vi "OAT Easy Resample Order Spectrum.vi"   [LabVIEW 2017]
doc: "Computes the order spectrum as power versus orders for <B>scaled signal [EU]</B>. You can use this polymorphic VI to compute the order spectrum for an analog tachometer signal or a digital tachometer signal. The data type you wire to the <B>analog tach signal</B> input determines the polymorphic instance to use."
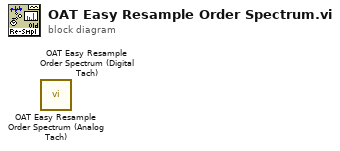
[diagram p0: block diagram]
diagram:
  n1 = call <vilib>:"OAT Easy Resample Order Spectrum (Analog Tach).vi"() -> ()  [unwired: 12 in, 4 out]
  n2 = call <vilib>:"OAT Easy Resample Order Spectrum (Digital Tach).vi"() -> ()  [unwired: 12 in, 4 out]
